vi "Write.vi"(8 "error in (no error)":errorcluster, 10 "Value":string, 11 "Class 1 in":refnum<class "csv.lvclass">) -> (0 "error out":errorcluster, 3 "Class 1 out":refnum<class "csv.lvclass">)   [LabVIEW 2021, in "Library.lvlib" / "csv.lvclass"]
uses:
  csv.lvclass
  csv.lvclass/csv.ctl
  <vilib>/Utility/file.llb/Write Delimited Spreadsheet (string).vi
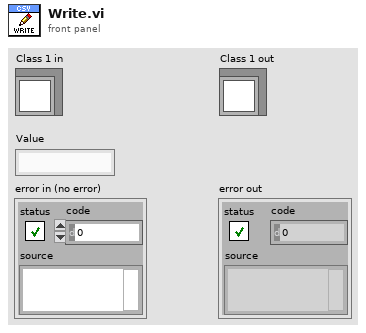
[diagram p1: front panel]
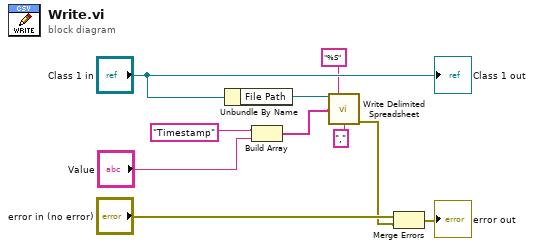
[diagram p0: block diagram]
diagram:
  n1 = Unbundle By Name("Class 1 in") -> ("File Path"=w8:path)
  n2 = Build Array("Timestamp", "Value") -> (w3:string[])
  n3 = call-poly <vilib>:"Write Delimited Spreadsheet.vi"("file path (dialog if empty)"=w8, "format (%s)"="%S" ("format (%.3f)"), "1D data"=w3, "delimiter (\\t)"="," ("delimiter (\\t)")) -> ("error out"=w1:errorcluster)  [unwired: 10 in, 1 out]
  n4 = Merge Errors("error in (no error)", w1) -> (→"error out":errorcluster)
  "Class 1 out" <- "Class 1 in"
